vi "FinalVI.vi"(10 "Numeric":dbl, 11 "Modbus Master in":refnum<class "Modbus Master.lvclass">) -> (0 "error out":errorcluster, 3 "Modbus Master out":refnum<class "Modbus Master.lvclass">)   [LabVIEW 2019]
uses:
  <vilib>/NI/Modbus Library/API/Master/Modbus Master.lvclass
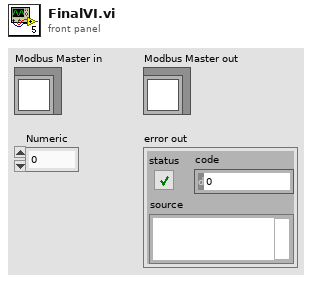
[diagram p1: front panel]
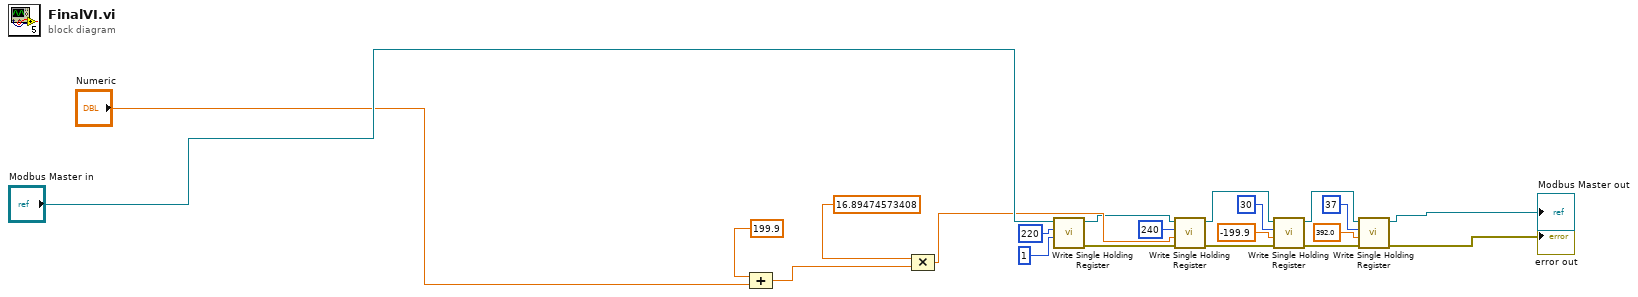
[diagram p0: block diagram]
diagram:
  n1 = Compound Arithmetic op=ADD(199.9 ("value"), "Numeric") -> (w3:dbl)
  n2 = Compound Arithmetic op=MULTIPLY(16.89474573408 ("value"), w3) -> (w20:dbl)
  n3 = call-dynamic "Write Single Holding Register.vi"("register to write"=u16 1, "address"=u16 220, "Modbus master in"="Modbus Master in") -> ("error out"=w19:errorcluster, "Modbus master out"=w18:refnum<class "Modbus Master.lvclass">)  [unwired: 7 in]
  n4 = call-dynamic "Write Single Holding Register.vi"("error in"=w19, "register to write"=w20, "address"=u16 240, "Modbus master in"=w18) -> ("error out"=w7:errorcluster, "Modbus master out"=w8:refnum<class "Modbus Master.lvclass">)  [unwired: 6 in]
  n5 = call-dynamic "Write Single Holding Register.vi"("error in"=w7, "register to write"=-199.9 ("value"), "address"=u16 30, "Modbus master in"=w8) -> ("error out"=w6:errorcluster, "Modbus master out"=w5:refnum<class "Modbus Master.lvclass">)  [unwired: 6 in]
  n6 = call-dynamic "Write Single Holding Register.vi"("error in"=w6, "register to write"=392.0 ("value"), "address"=u16 37, "Modbus master in"=w5) -> ("error out"=→"error out":errorcluster, "Modbus master out"=→"Modbus Master out":refnum<class "Modbus Master.lvclass">)  [unwired: 6 in]
